vi "数据查询_报警信息.vi"() -> ()   [LabVIEW 2016]
uses:
  <vilib>/Utility/miscctls.llb/LVRowAndColumnUnsignedTypeDef.ctl
  <vilib>/Utility/miscctls.llb/LVPositionTypeDef.ctl
  <vilib>/Utility/miscctls.llb/LVPointTypeDef.ctl
  <userlib>/_OpenG.lib/array/array.llb/Sort 2D Array (String)__ogtk.vi
  <userlib>/_OpenG.lib/array/array.llb/Sort 1D Array (I32)__ogtk.vi
panel:
  in  "查询触发":bool
  out "显示项":string[](array[string])
  out "确定查询":bool
  out "condition":string
  in  "数据列表选择框":string(xcontrol)
  in  "导出":bool
  in  "条件筛选":bool
  in  "数据表":T1
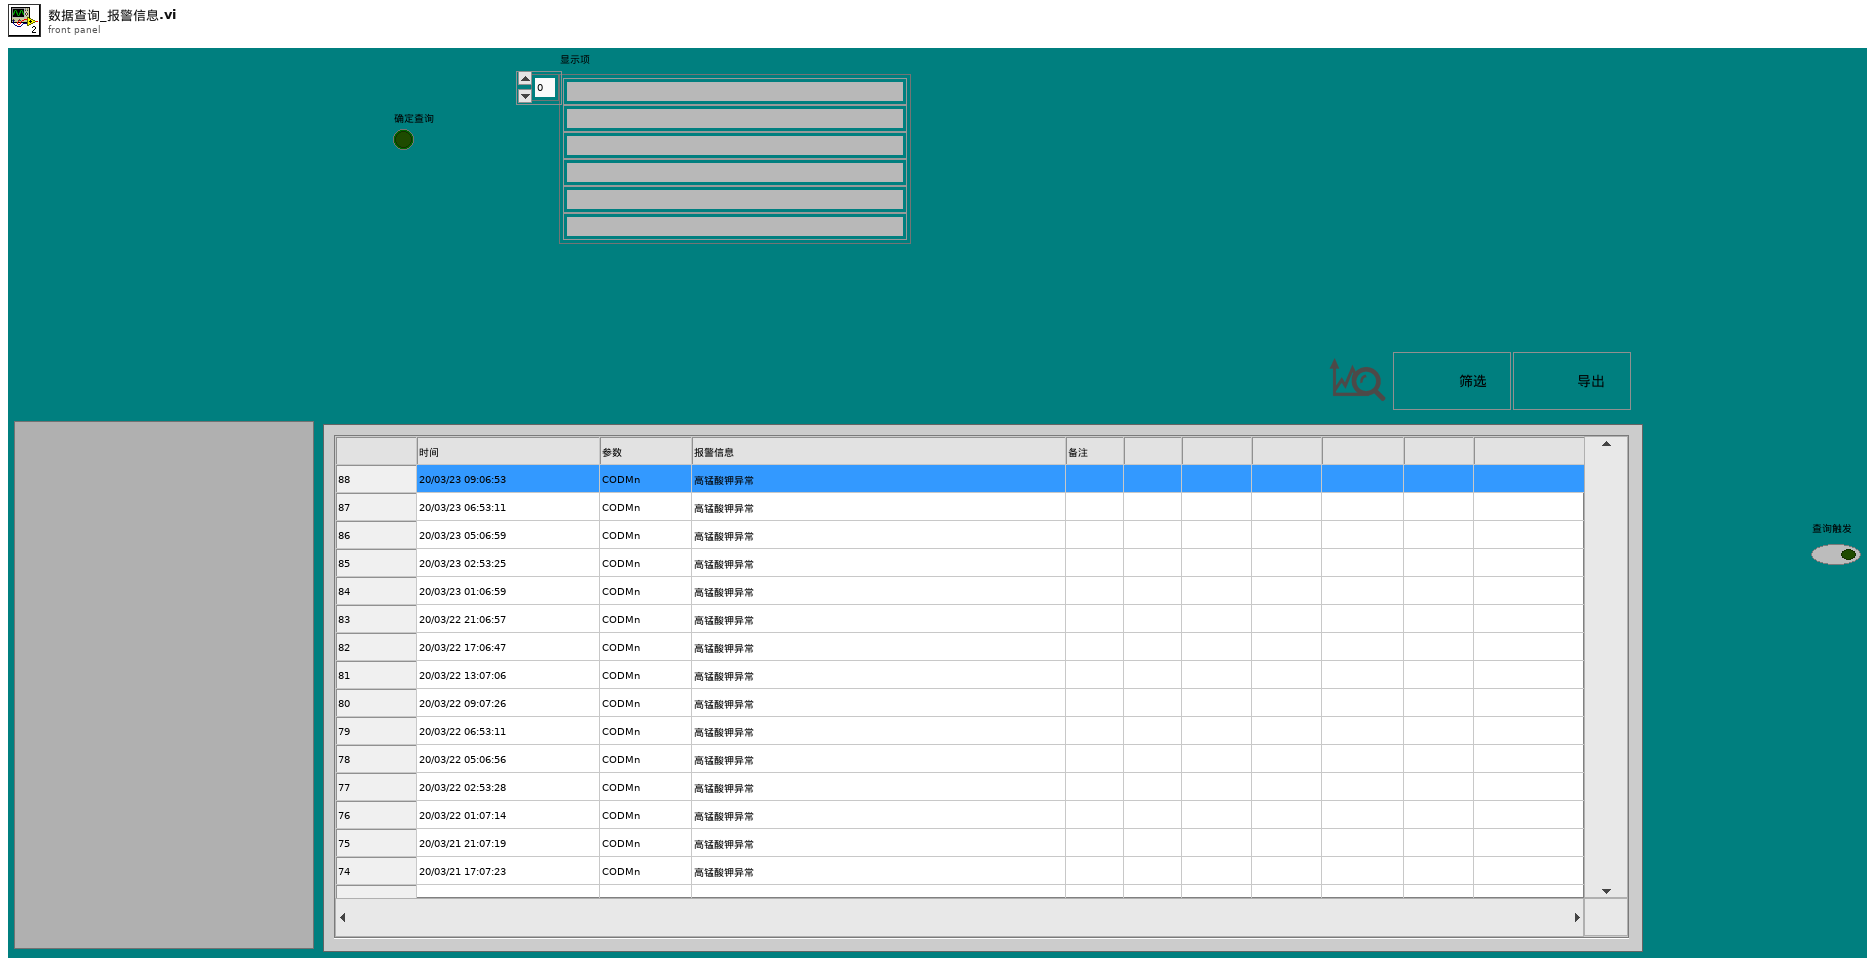
[diagram p1: front panel]
types:
  T1 = typedef "数据查询大列表框.ctl" = i32
  T2 = typedef "LVPositionTypeDef.ctl" = cluster{"Left":i32, "Top":i32}
  T3 = typedef "LVRowAndColumnUnsignedTypeDef.ctl" = cluster{"Row":u32, "Column":u32}
  T4 = typedef "LVPointTypeDef.ctl" = cluster{"Horizontal":i16, "Vertical":i16}
  T5 = enum8{"Enabled", "Disabled", "Disabled and Grayed Out"}
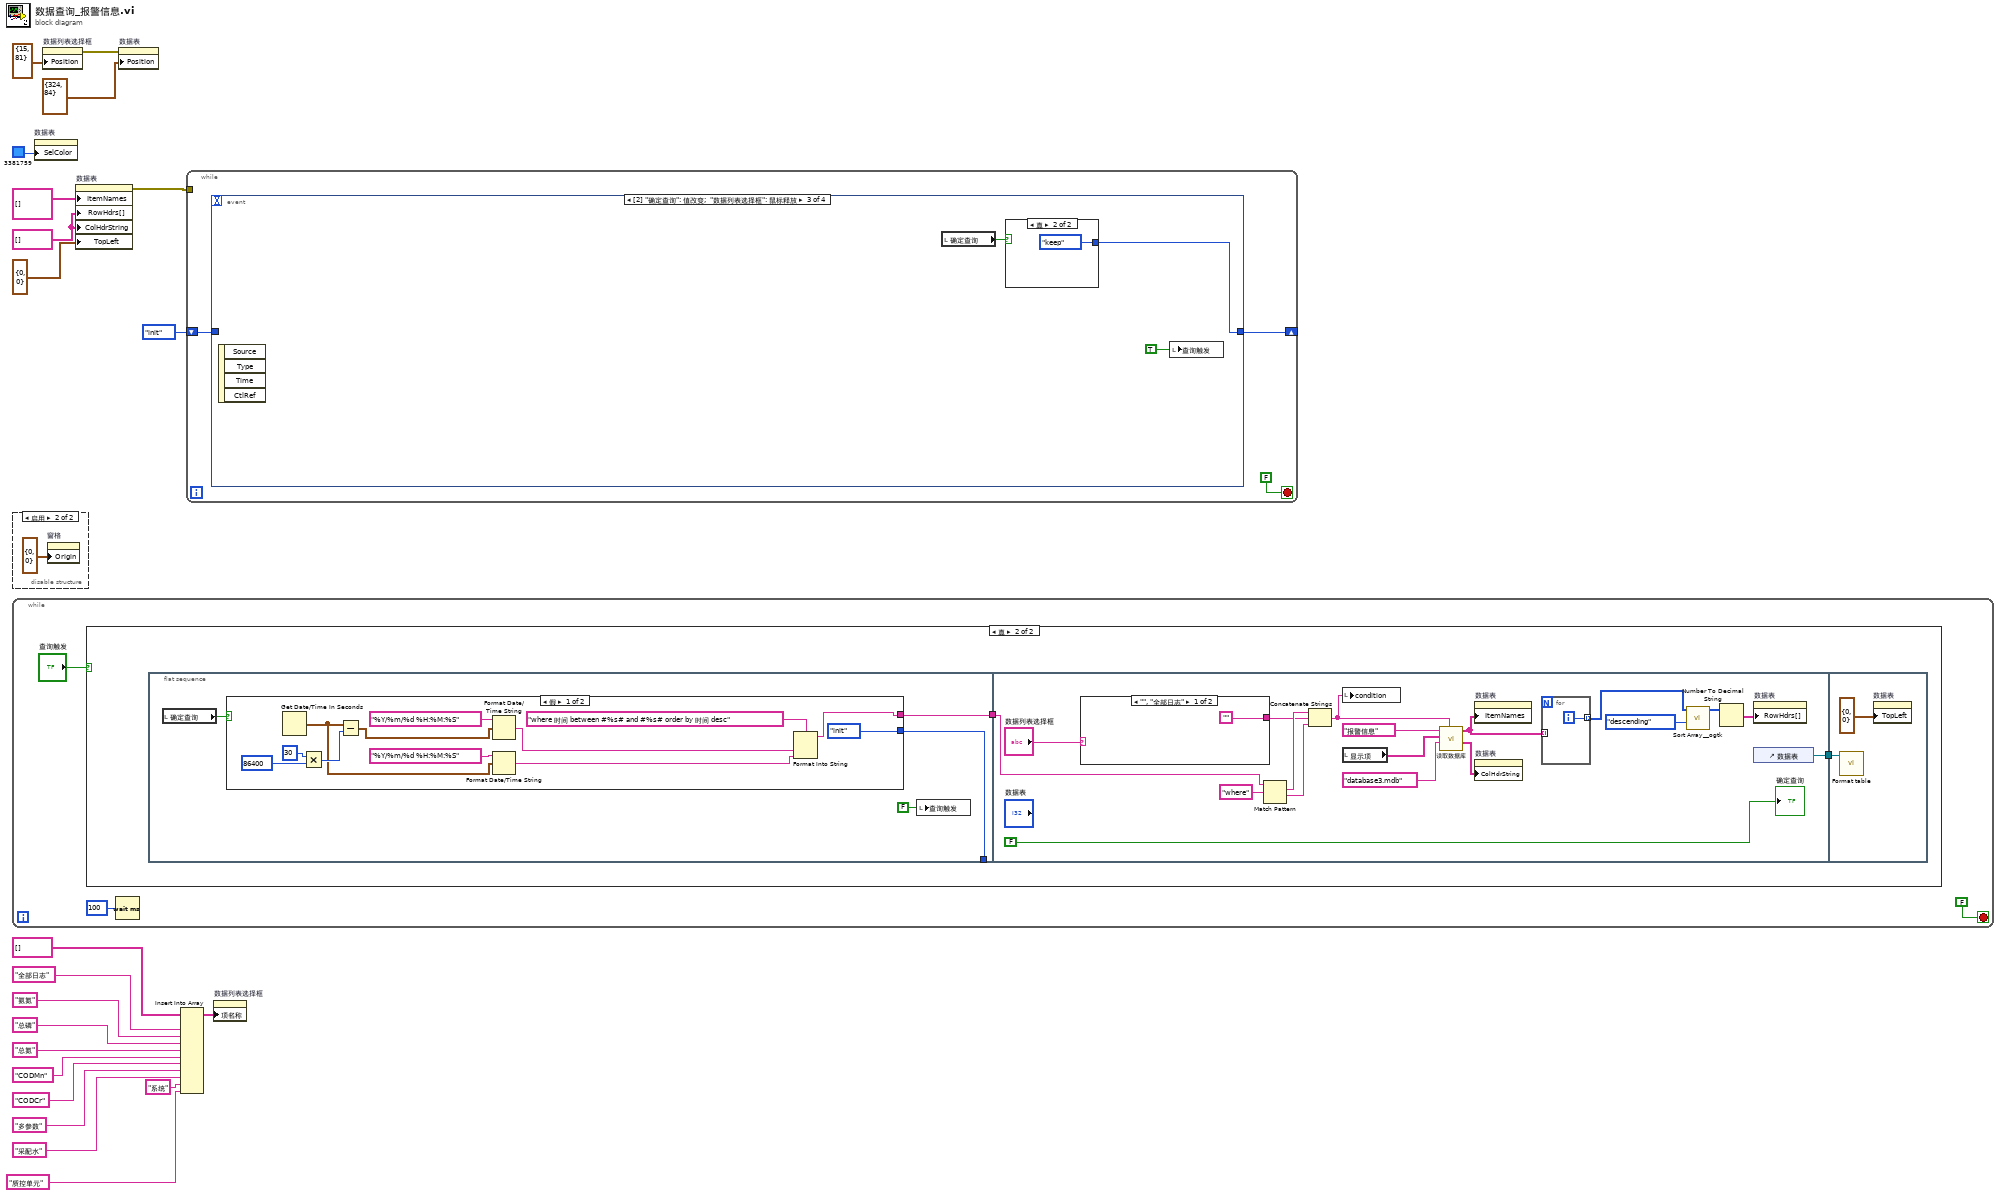
[diagram p0: block diagram]
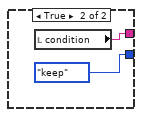
[diagram p3: hidden frame]
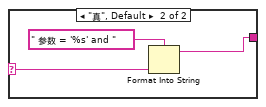
[diagram p4: hidden frame]
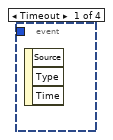
[diagram p5: hidden frame]
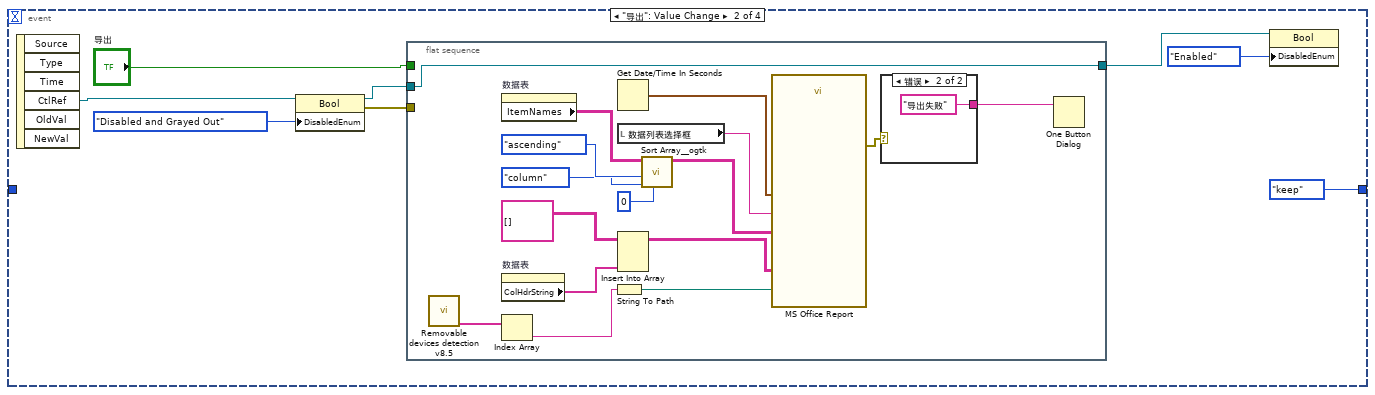
[diagram p6: hidden frame]
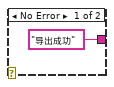
[diagram p7: hidden frame]
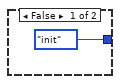
[diagram p8: hidden frame]
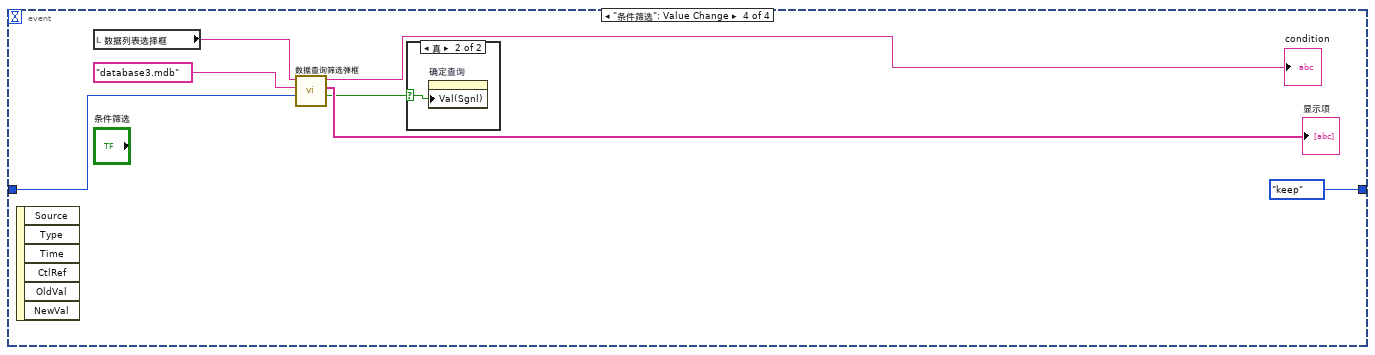
[diagram p9: hidden frame]
diagram:
  w9 = string[] [] ("行首字符串[]")
  n1 = disable-structure shown="启用" {
    frame Disabled {
    }
    frame Enabled {
      n2 = property on="窗格" class="Pane"("Origin"=T4 {"Horizontal"=0, "Vertical"=0} ("原点")) -> ()  [unwired: 2 in, 2 out]
    }
  }
  n3 = while {
    stop <- FALSE stop-if-true
    n4 = case shown="真" "查询触发" {
      frame False {
      }
      frame True {
        n5 = flat-sequence {
          tunnel: [w30] -> w27
          tunnel: [w29] -> _
          tunnel: [w55] -> w26
          tunnel: w27 -> [w50]
          tunnel: w26 -> [w69]
          frame #0 {
            n6 = local read "确定查询"() -> (w31:bool)
            n7 = case shown="假" w31 {
              tunnel: [w34 w44] -> w30
              tunnel: [enum16{"init", "keep"}."init" ("是否初始化") enum16{"init", "keep"}."keep" ("是否初始化")] -> w29
              frame False {
                n8 = Get Date/Time In Seconds() -> (seconds since 1Jan1904=w32:timestamp)
                n9 = Multiply(x=30, y=86400) -> (x*y=w35:i32)
                n10 = Subtract(x=w32, y=w35) -> (x-y=w40:timestamp)
                n11 = Format Date/Time String(time format string (%c)="%Y/%m/%d %H:%M:%S" ("时间格式字符串(%c)"), seconds (now)=w40) -> (date/time string=w42:string)  [unwired: 1 in]
                n12 = Format Date/Time String(time format string (%c)="%Y/%m/%d %H:%M:%S" ("时间格式字符串(%c)"), seconds (now)=w32) -> (date/time string=w43:string)  [unwired: 1 in]
                n13 = Format Into String(format string="where 时间 between #%s# and #%s# order by 时间 desc", w42, w43) -> (resulting string=w34:string)  [unwired: 2 in, 1 out]
              }
              frame True {
                n14 = local read "condition"() -> (w44:string)
              }
            }
            n15 = local write "查询触发"(FALSE ("查询触发")) -> ()
          }
          frame #1 {
            n16 = case shown="\"\", \"全部日志\"" "数据列表选择框" {
              selector: "数据列表选择框" -> [_ w66]
              tunnel: ["" w65] -> w49
              frame "", "全部日志" {
              }
              frame "真", Default {
                n17 = Format Into String(format string=" 参数 = '%s' and " ("condition"), w66) -> (resulting string=w65:string)  [unwired: 2 in, 1 out]
              }
            }
            n18 = Match Pattern(string=w50, regular expression="where") -> (match substring=w52:string, after substring=w51:string)  [unwired: 1 in, 2 out]
            n19 = Concatenate Strings(w52, w49, w51) -> (w48:string)
            n20 = local write "condition"(w48) -> ()
            n21 = local read "显示项"() -> (w46:string[])
            n22 = call "读取数据库.vi"("condition"=w48, "database"="database3.mdb", "显示项"=w46, "组合框"="报警信息") -> ("columns"=w63:string[], "表格"=w58:string[][])  [unwired: 4 in, 2 out]
            n23 = property on="数据表" class="MCListbox (严格)"("ItemNames"=w58) -> ()  [unwired: 2 in, 2 out]
            n24 = property on="数据表" class="MCListbox (严格)"("ColHdrString"=w63) -> ()  [unwired: 2 in, 2 out]
            n25 = for {
              tunnel: w58 -> [_] mode=indexing
              tunnel: [w68] -> w62 mode=indexing
              i -> [w68]
            }
            n26 = call-poly <userlib>:"Sort Array__ogtk.vi"("Order"=enum16{"ascending", "descending"}."descending", "Array in"=w62) -> ("Sorted Array out"=w57:i32[])  [unwired: 8 in, 1 out]
            n27 = Number To Decimal String(number=w57) -> (decimal integer string=w61:string[])  [unwired: 1 in]
            n28 = property on="数据表" class="MCListbox (严格)"("RowHdrs[]"=w61) -> ()  [unwired: 2 in, 2 out]
            n29 = control-ref of="数据表"() -> (w55:refnum<vi>)
            "确定查询" <- FALSE ("确定查询")
          }
          frame #2 {
            n30 = call "Format table.vi"("Table输入"=w69) -> ()  [unwired: 11 in]
            n31 = property on="数据表" class="MCListbox (严格)"("TopLeft"=T3 {"Row"=0, "Column"=0} ("索引值")) -> ()  [unwired: 2 in, 2 out]
          }
        }
      }
    }
    n32 = Wait (ms)(milliseconds to wait=u32 100 ("等待时间（毫秒）")) -> ()  [unwired: 1 out]
  }
  n33 = property on="数据表" class="MCListbox (严格)"("SelColor"=u32 3381759) -> ()  [unwired: 2 in, 2 out]
  n34 = property on="数据列表选择框" class="数据列表选择框 (严格)"("Position"=T2 {"Left"=15, "Top"=81} ("位置")) -> (error out=w2:errorcluster)  [unwired: 2 in, 1 out]
  n35 = property on="数据表" class="MCListbox (严格)"("ItemNames"=string[][] [] ("项名"), "RowHdrs[]"=w9, "ColHdrString"=w9, "TopLeft"=T3 {"Row"=0, "Column"=0} ("左上可见单元格")) -> (error out=w11:errorcluster)  [unwired: 2 in, 1 out]
  n36 = property on="数据表" class="MCListbox (严格)"(error in=w2, "Position"=T2 {"Left"=324, "Top"=84} ("位置")) -> ()  [unwired: 1 in, 2 out]
  n37 = Insert Into Array(array=string[] [], new element #1="全部日志" ("新元素/子数组"), new element #2="氨氮" ("新元素/子数组"), new element #3="总磷" ("新元素/子数组"), new element #4="总氮" ("新元素/子数组"), new element #5="CODMn" ("新元素/子数组"), new element #6="CODCr" ("新元素/子数组"), new element #7="多参数" ("新元素/子数组"), new element #8="采配水" ("新元素/子数组"), new element #9="系统" ("新元素/子数组"), new element #10="质控单元" ("新元素/子数组")) -> (w7:string[])  [unwired: 1 in]
  n38 = while {
    tunnel: w11 -> [_]
    shift-right: [w71] -> _
    shift-left: enum16{"init", "keep"}."init" ("是否初始化") -> [w72]
    stop <- FALSE stop-if-true
    n39 = event shown="[2] \"确定查询\": 值改变;  \"数据列表选择框\": 鼠标释放" {
      selector: _ -> [_ _ _ _]
      dyn-events: _ -> [_ _ _ _]
      timeout: _ -> [_ _ _ _]
      tunnel: w72 -> [_ _ _ w106]
      tunnel: [_ enum16{"init", "keep"}."keep" ("是否初始化") w101 enum16{"init", "keep"}."keep" ("是否初始化")] -> w71
      event Timeout {
        n40 = event-data() -> ()  [unwired: 1 in, 3 out]
      }
      event "导出": Value Change {
        n41 = event-data() -> ("CtlRef"=w75:refnum<vi>)  [unwired: 1 in, 5 out]
        n42 = property class="Bool"(reference=w75, "DisabledEnum"=T5."Disabled and Grayed Out" ("禁用")) -> (reference out=w79:refnum<vi>, error out=w80:errorcluster)  [unwired: 1 in]
        n43 = flat-sequence {
          tunnel: w80 -> [_]
          tunnel: [w91] -> w78
          tunnel: w79 -> [w91]
          tunnel: "导出" -> [_]
          frame #0 {
            n44 = call "Removable devices detection v8.5.vi"() -> ("Removable"=w88:string[])  [unwired: 4 out]
            n45 = property on="数据表" class="MCListbox (严格)"() -> ("ItemNames"=w82:string[][])  [unwired: 2 in, 2 out]
            n46 = property on="数据表" class="MCListbox (严格)"() -> ("ColHdrString"=w84:string[])  [unwired: 2 in, 2 out]
            n47 = Index Array(array=w88) -> (element=w87:string)  [unwired: 1 in]
            n48 = String To Path(string=w87) -> (path=w86:path)
            n49 = Get Date/Time In Seconds() -> (seconds since 1Jan1904=w97:timestamp)
            n50 = local read "数据列表选择框"() -> (w92:string)
            n51 = Insert Into Array(array=string[][] [], new element=w84) -> (w83:string[][])  [unwired: 2 in]
            n52 = call-poly <userlib>:"Sort Array__ogtk.vi"("Column/Row to Sort By"=u32 0, "Sort By in"=enum16{"row", "column"}."column", "Order"=enum16{"ascending", "descending"}."ascending", "Array in"=w82) -> ("Sorted Array out"=w96:string[][])  [unwired: 4 in, 3 out]
            n53 = call "MS Office Report"("Path to Save Report"=w86, "导出日期"=w97, "监测参数"=w92, "数据输入"=w96, "字段定义"=w83) -> ("error out"=w90:errorcluster)  [unwired: 21 in, 1 out]
            n54 = case shown="错误" w90 {
              tunnel: ["导出成功" ("消息") "导出失败" ("消息")] -> w89
              frame No Error {
              }
              frame Error {
              }
            }
            n55 = One Button Dialog(message=w89) -> ()  [unwired: 1 in, 1 out]
          }
        }
        n56 = property class="Bool"(reference=w78, "DisabledEnum"=T5."Enabled" ("禁用")) -> ()  [unwired: 1 in, 2 out]
      }
      event "确定查询": Value Change; "数据列表选择框": Mouse Up {
        n57 = event-data() -> ()  [unwired: 1 in, 4 out]
        n58 = local read "确定查询"() -> (w102:bool)
        n59 = case shown="真" w102 {
          tunnel: [enum16{"init", "keep"}."init" ("是否初始化") enum16{"init", "keep"}."keep" ("是否初始化")] -> w101
          frame False {
          }
          frame True {
          }
        }
        n60 = local write "查询触发"(TRUE ("查询触发")) -> ()
      }
      event "条件筛选": Value Change {
        n61 = event-data() -> ()  [unwired: 1 in, 6 out]
        n62 = local read "数据列表选择框"() -> (w107:string)
        n63 = call "数据查询筛选弹框.vi"("是否初始化"=w106, "database"="database3.mdb", "table"=w107) -> ("确定输出"=w108:bool, "显示项"=→"显示项":string[], "condition"=→"condition":string)  [unwired: 5 in, 1 out]
        n64 = case shown="真" w108 {
          selector: w108 -> [_ w112]
          frame False {
          }
          frame True {
            n65 = property on="确定查询" class="Bool (严格)"("Val(Sgnl)"=w112) -> ()  [unwired: 2 in, 2 out]
          }
        }
      }
    }
  }
  n66 = property on="数据列表选择框" class="数据列表选择框 (严格)"("项名称"=w7) -> ()  [unwired: 2 in, 2 out]
